vi "GF_AgilentDownloadAll.vi"(4 "Error In":errorcluster, 5 "Agilent Download":bool=TRUE, 6 "Agilent Cluster In":T1={"Trig?"=FALSE, "VISA session"="", "Setup to Load"="CH1", "Timeout (ms)"=10000, "Desired Samp"=enum."100", "Captured Samp"=0, "Desired Channels"=[]}, 7 "File Path":path) -> (0 "error out":errorcluster, 2 "Agilent Cluster Out":T1={"Trig?"=FALSE, "VISA session"="", "Setup to Load"="CH1", "Timeout (ms)"=10000, "Desired Samp"=enum."100", "Captured Samp"=0, "Desired Channels"=[]}, 3 "Agilent Scintillator Scope Graph":waveform(dbl)[](graph))   [LabVIEW 2020]
uses:
  AgilentControl.ctl
  Channel Config.ctl
  <vilib>/Waveform/WDTOps.llb/WDT Number of Waveform Samples DBL.vi
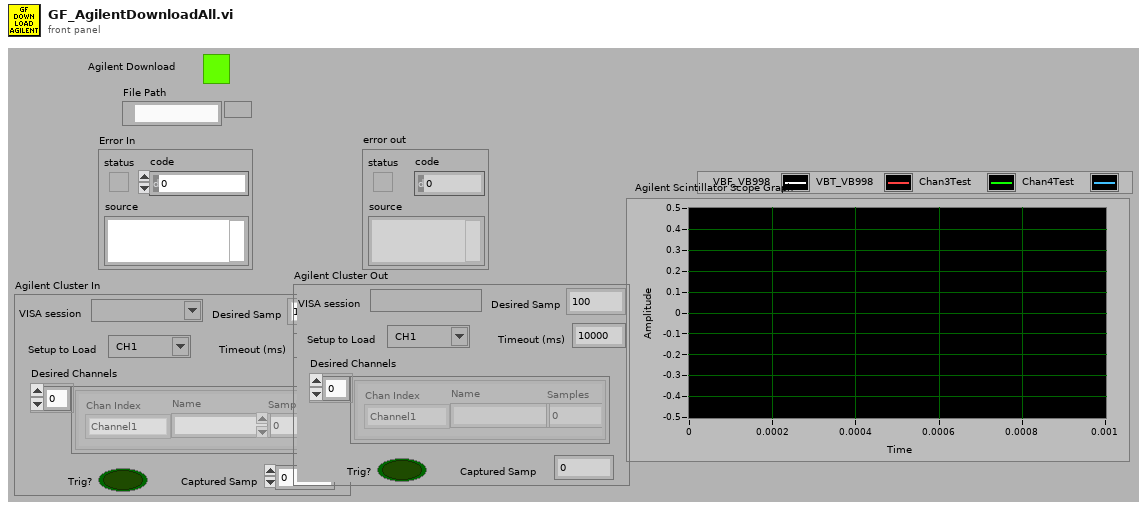
[diagram p1: front panel]
types:
  T1 = typedef "AgilentControl.ctl" = cluster{"Trig?":bool, "VISA session":refnum<visa-resource-name>, "Setup to Load":string, "Timeout (ms)":u32, "Desired Samp":enum32{"100", "250", "500", "1000", "2000", "5000", "10000", "20000", "50000", "100000", "200000", "500000", "1000000", "2000000", "4000000", "8000000"}, "Captured Samp":i32, "Desired Channels":T2[]}
  T2 = typedef "Channel Config.ctl" = cluster{"Chan Index":enum16{"Channel1", "Channel2", "Channel3", "Channel4", "MATH"}, "Name":string, "Samples":i32}
  T3 = enum16{"Channel1", "Channel2", "Channel3", "Channel4", "MATH"}
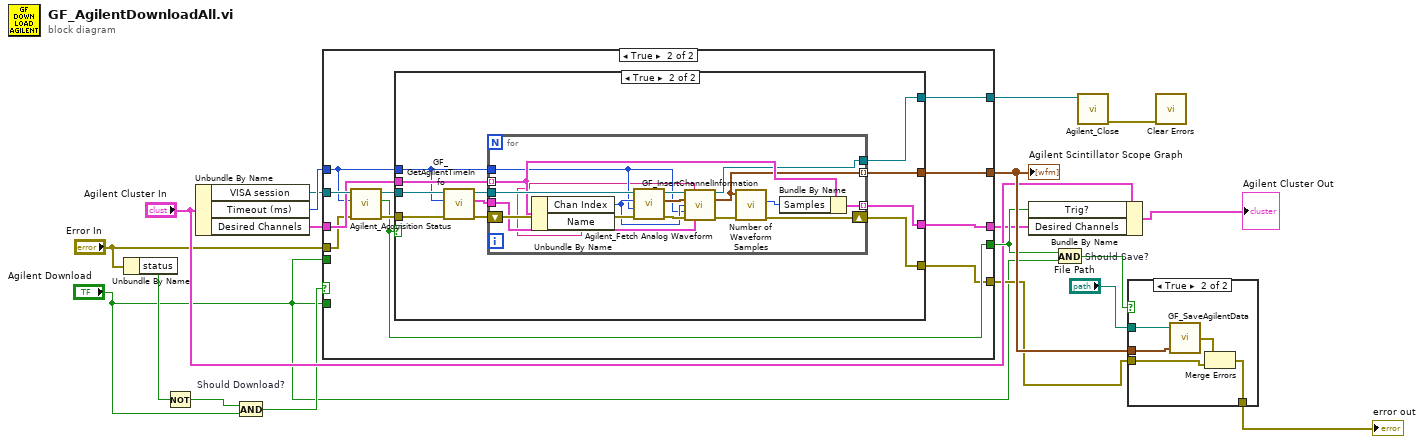
[diagram p0: block diagram]
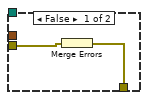
[diagram p2: hidden frame]
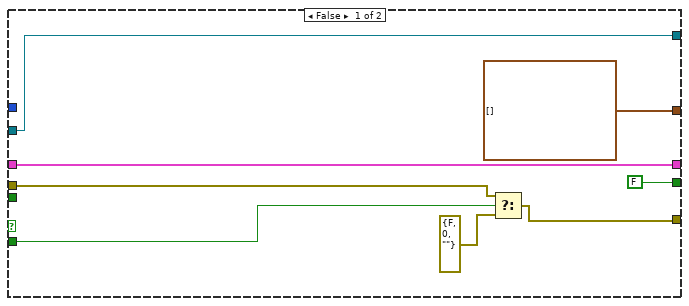
[diagram p3: hidden frame]
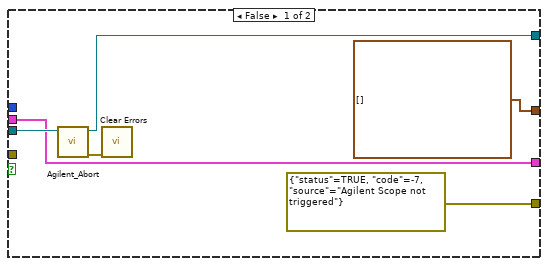
[diagram p4: hidden frame]
diagram:
  n1 = Unbundle By Name("Error In") -> ("status"=w4:bool)
  n2 = Not(x=w4) -> (.not. x?=w3:bool)
  n3 = Unbundle By Name("Agilent Cluster In") -> ("VISA session"=w16:refnum<visa-resource-name>, "Timeout (ms)"=w17:u32, "Desired Channels"=w18:T2[])
  n4 = And "Should Download?"(x=w3, y="Agilent Download") -> (x .and. y?=w2:bool)
  n5 = case shown="True" w2 {
    tunnel: [w26 w37] -> w14
    tunnel: [waveform(dbl)[] [] w36] -> w13
    tunnel: [w20 w30] -> w6
    tunnel: w16 -> [w26 w34]
    tunnel: "Error In" -> [w22 w28]
    tunnel: w17 -> [_ w32]
    tunnel: w18 -> [w24 w33]
    tunnel: [FALSE ("Acquisition Complete?") w31] -> w11
    tunnel: "Agilent Download" -> [_ _]
    tunnel: [w24 w29] -> w7
    tunnel: "Agilent Download" -> [w23 _]
    frame False {
      n6 = Select(t=w22, s=w23, f=errorcluster {"status"=FALSE, "code"=0, "source"=""}) -> (s? t:f=w20:errorcluster)
    }
    frame True {
      n7 = call "Agilent_Acquisition Status.vi"("error in (no error)"=w28, "Timeout (10000 ms)"=w32, "VISA resource name"=w34) -> ("error out"=w35:errorcluster, "Acquisition Complete?"=w31:bool, "VISA resource name out"=w38:refnum<visa-resource-name>)  [unwired: 6 in]
      n8 = case shown="True" w31 {
        tunnel: w38 -> [w43 w48]
        tunnel: w35 -> [_ w47]
        tunnel: w33 -> [w40 w55]
        tunnel: [w42 w54] -> w37
        tunnel: [errorcluster {"status"=TRUE, "code"=-7, "source"="Agilent Scope not triggered"} ("error out") w53] -> w30
        tunnel: [waveform(dbl)[] [] w52] -> w36
        tunnel: w32 -> [_ w46]
        tunnel: [w40 w51] -> w29
        frame False {
          n9 = call "Agilent_Abort.vi"("VISA resource name"=w43) -> ("error out"=w41:errorcluster, "VISA resource name out"=w42:refnum<visa-resource-name>)  [unwired: 9 in]
          n10 = call <vilib>:"Clear Errors.vi"("error in (no error)"=w41) -> ()  [unwired: 5 in, 2 out]
        }
        frame True {
          n11 = call "GF_GetAgilentTimeInfo.vi"("error in (no error)"=w47, "Timeout (10000 ms)"=w46, "VISA resource name"=w48) -> ("error out"=w50:errorcluster, "Timing Info"=w45:cluster{"Name":string, "Value":string}[], "VISA resource name out"=w49:refnum<visa-resource-name>)  [unwired: 6 in]
          n12 = for {
            tunnel: w49 -> [w71]
            tunnel: w55 -> [w68] mode=indexing
            tunnel: [w60] -> w52 mode=indexing
            tunnel: [w65] -> w54
            tunnel: w46 -> [w58]
            tunnel: [w67] -> w51 mode=indexing
            tunnel: w45 -> [w57]
            shift-right: [w69] -> w53
            shift-left: w50 -> [w70]
            n13 = Unbundle By Name(w68) -> ("Chan Index"=w59:T3, "Name"=w56:string)
            n14 = call "Agilent_Fetch Analog Waveform.vi"("error in (no error)"=w70, "Timeout (10000 ms)"=w58, "Source (0: Channel 1)"=w59, "VISA resource name"=w71) -> ("error out"=w62:errorcluster, "Waveform Data"=w63:waveform(dbl), "VISA resource name out"=w64:refnum<visa-resource-name>)  [unwired: 5 in]
            n15 = call "GF_InsertChannelInformation.vi"("VISA resource name"=w64, "Channel Name"=w56, "Waveform In"=w63, "Source (0: Channel 1)"=w59, "Timeout (10000 ms)"=w58, "error in (no error)"=w62, "Timing Info"=w57) -> ("VISA resource name out"=w65:refnum<visa-resource-name>, "waveform out"=w60:waveform(dbl), "error out"=w61:errorcluster)  [unwired: 6 in]
            n16 = call-poly <vilib>:"Number of Waveform Samples.vi"("error in (no error)"=w61, "waveform in"=w60) -> ("error out"=w69:errorcluster, "number of samples"=w66:i32)  [unwired: 7 in, 1 out]
            n17 = Bundle By Name(cluster=w68, "Samples"=w66) -> (w67:T2)
          }
        }
      }
    }
  }
  "Agilent Scintillator Scope Graph" <- w13
  n18 = Bundle By Name(cluster="Agilent Cluster In", "Trig?"=w11, "Desired Channels"=w7) -> (→"Agilent Cluster Out":T1)
  n19 = And "Should Save?"(x=w11, y="Agilent Download") -> (x .and. y?=w12:bool)
  n20 = call "Agilent_Close.vi"("VISA resource name"=w14) -> ("error out"=w15:errorcluster)  [unwired: 10 in]
  n21 = case shown="True" w12 {
    tunnel: w13 -> [_ w78]
    tunnel: "File Path" -> [_ w77]
    tunnel: w6 -> [w73 w75]
    tunnel: [w72 w74] -> w5
    frame False {
      n22 = Merge Errors(w73) -> (w72:errorcluster)
    }
    frame True {
      n23 = call "GF_SaveAgilentData.vi"("Agilent Scintillator Scope Graph"=w78, "Base Path"=w77) -> ("error out"=w76:errorcluster)  [unwired: 1 in]
      n24 = Merge Errors(w76, w75) -> (w74:errorcluster)
    }
  }
  "error out" <- w5
  n25 = call <vilib>:"Clear Errors.vi"("error in (no error)"=w15) -> ()  [unwired: 5 in, 2 out]
